vi "refregirator.final.vi"() -> ()   [LabVIEW 2022 SP3]
uses:
  <vilib>/DAQmx/miscellaneous.llb/DAQmx Fill In Error Info.vi
  <vilib>/DAQmx/read.llb/DAQmx Read (Digital Bool 1Line 1Point).vi
  <vilib>/DAQmx/write.llb/DAQmx Write (Digital Bool 1Line 1Point).vi
  <vilib>/DAQmx/read.llb/DAQmx Read (Analog 1D DBL NChan 1Samp).vi
  <vilib>/DAQmx/create/channels.llb/DAQmx Create Channel (DI-Digital Input).vi
  <vilib>/DAQmx/create/channels.llb/DAQmx Create Channel (DO-Digital Output).vi
  <vilib>/DAQmx/create/channels.llb/DAQmx Create Channel (AI-Voltage-Basic).vi
panel:
  out "Cool":bool
  in  "Door Input":tag
  out "Door closed":bool
  in  "Digital Output(Fan)":tag
  out "State":string
  out "Numerical State":dbl
  out "Thermistor temparature":dbl
  out "Outdoor temparature":dbl
  out "Set temparature":dbl
  out "Inside temparature":dbl(knob) scale=0.0..40.0
  out "Outdoor temparature(Celsius)":dbl(knob) scale=0.0..50.0
  in  "stop":bool
  out "Set temparature(Celsius)":dbl(knob) scale=10.0..50.0
  in  "Analog Inputs (Sensors)":tag
  # "Smart Thermo Electric Cooler"
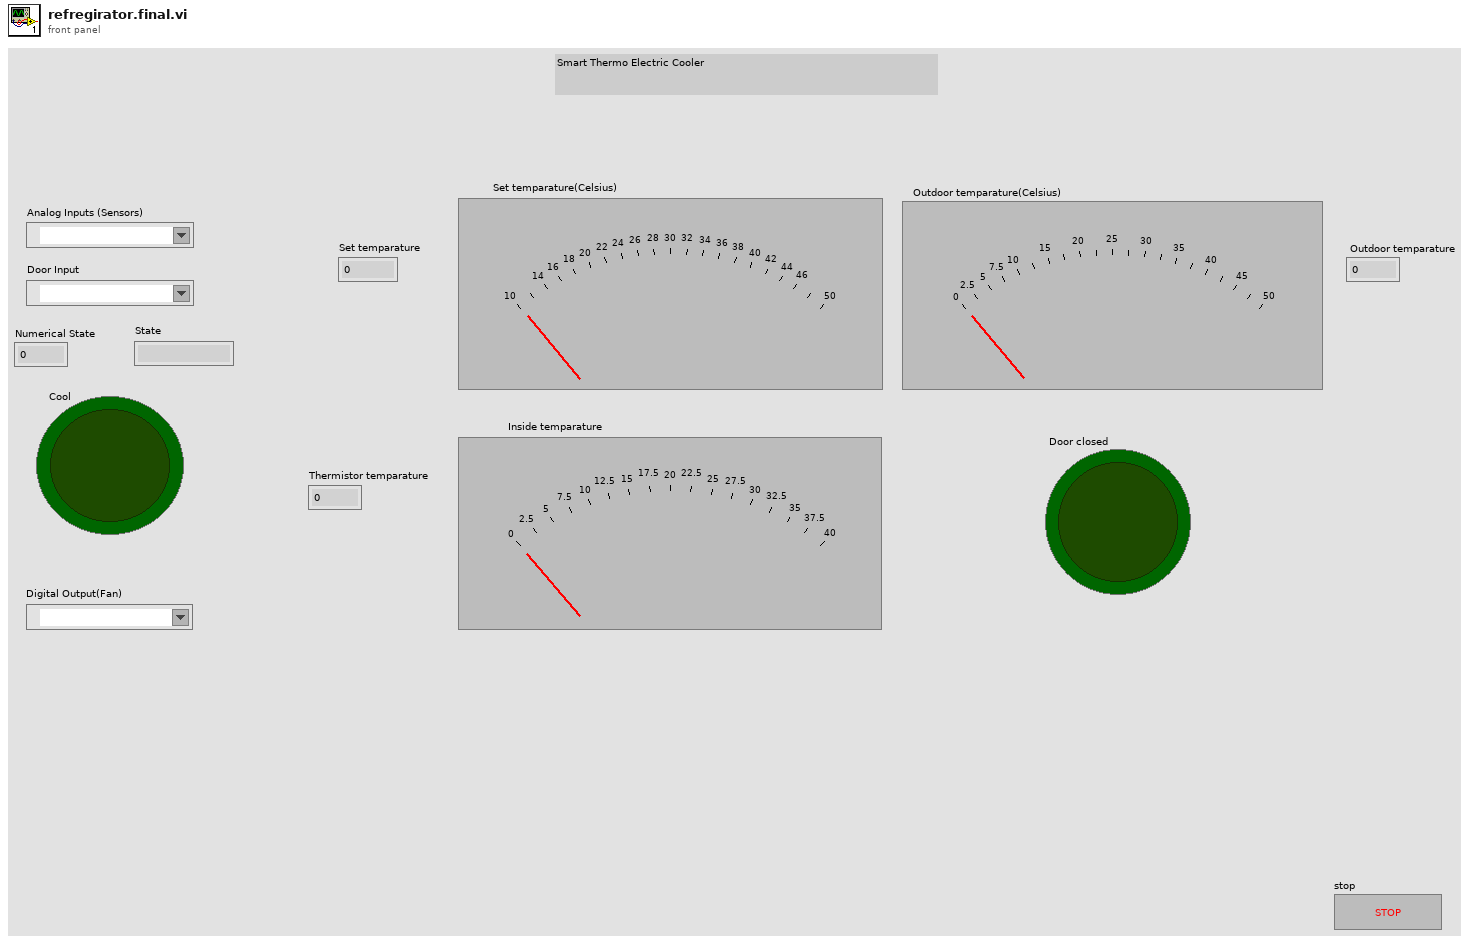
[diagram p1: front panel]
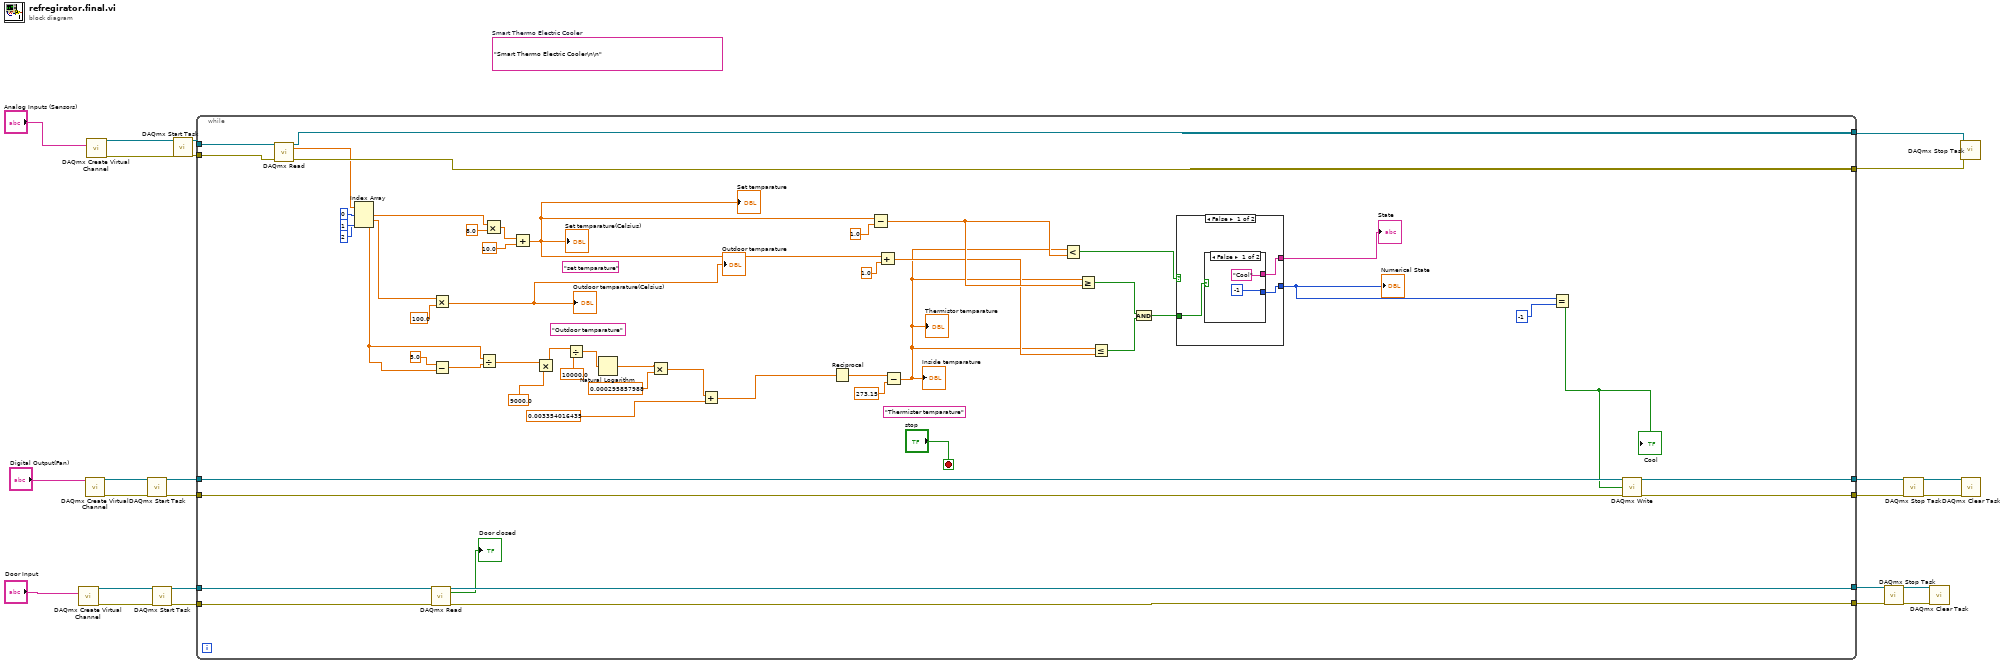
[diagram p0: block diagram]
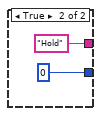
[diagram p2: hidden frame]
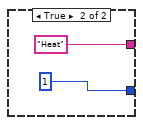
[diagram p3: hidden frame]
diagram:
  (unwired) "Smart Thermo Electric Cooler\n\n"  # Smart Thermo Electric Cooler
  n1 = call-poly <vilib>:"DAQmx Create Virtual Channel.vi"("lines"="Door Input") -> ("task out"=w9:refnum<k21>, "error out"=w8:errorcluster)  [unwired: 13 in]
  n2 = call-poly <vilib>:"DAQmx Create Virtual Channel.vi"("lines"="Digital Output(Fan)") -> ("task out"=w18:refnum<k21>, "error out"=w17:errorcluster)  [unwired: 13 in]
  n3 = call-poly <vilib>:"DAQmx Create Virtual Channel.vi"("physical channels"="Analog Inputs (Sensors)") -> ("task out"=w24:refnum<k21>, "error out"=w23:errorcluster)  [unwired: 13 in]
  n4 = call <vilib>:"DAQmx Start Task.vi"("task/channels in"=w18, "error in"=w17) -> ("task out"=w16:refnum<k21>, "error out"=w15:errorcluster)  [unwired: 12 in]
  n5 = call <vilib>:"DAQmx Start Task.vi"("task/channels in"=w9, "error in"=w8) -> ("task out"=w7:refnum<k21>, "error out"=w6:errorcluster)  [unwired: 12 in]
  n6 = call <vilib>:"DAQmx Start Task.vi"("task/channels in"=w24, "error in"=w23) -> ("task out"=w22:refnum<k21>, "error out"=w21:errorcluster)  [unwired: 12 in]
  n7 = while {
    tunnel: w22 -> [w79]
    tunnel: w21 -> [w78]
    tunnel: [w77] -> w20
    tunnel: [w76] -> w19
    tunnel: w16 -> [w44]
    tunnel: w15 -> [w43]
    tunnel: [w42] -> w14
    tunnel: [w41] -> w13
    tunnel: w7 -> [w33]
    tunnel: w6 -> [w32]
    tunnel: [w31] -> w3
    tunnel: [w30] -> w2
    stop <- "stop" stop-if-true
    (unwired) "Outdoor temparature"
    (unwired) "set temparature"
    (unwired) "Thermister temparature"
    n8 = call-poly <vilib>:"DAQmx Read.vi"("task/channels in"=w79, "error in"=w78) -> ("task out"=w77:refnum<k21>, "data"=w71:dbl[], "error out"=w76:errorcluster)  [unwired: 11 in]
    n9 = Index Array(array=w71, index #1=0 ("index"), index #2=1 ("index"), index #3=2 ("index")) -> (element #1=w67:dbl, element #2=w40:dbl, element #3=w59:dbl)
    n10 = call-poly <vilib>:"DAQmx Read.vi"("task/channels in"=w33, "error in"=w32) -> ("task out"=w31:refnum<k21>, "data"=→"Door closed":bool, "error out"=w30:errorcluster)  [unwired: 11 in]
    n11 = Multiply(x=w40, y=100.0) -> (x*y=→"Outdoor temparature(Celsius)" →"Outdoor temparature":dbl)
    n12 = Subtract(x=5.0 ("y"), y=w59) -> (x-y=w58:dbl)
    n13 = Divide(x=w59, y=w58) -> (x/y=w66:dbl)
    n14 = Multiply(x=w67, y=8.0) -> (x*y=w74:dbl)
    n15 = Add(x=w74, y=10.0) -> (x+y=w28:dbl)
    "Set temparature(Celsius)" <- w28
    "Set temparature" <- w28
    n16 = Multiply(x=w66, y=9000.0) -> (x*y=w34:dbl)
    n17 = Divide(x=w34, y=10000.0) -> (x/y=w36:dbl)
    n18 = Natural Logarithm(1:w36) -> (0:w62:dbl)
    n19 = Multiply(x=w62, y=0.000295857988) -> (x*y=w61:dbl)
    n20 = Add(x=w61, y=0.003354016435) -> (x+y=w35:dbl)
    n21 = Reciprocal(x=w35) -> (1/x=w57:dbl)
    n22 = Subtract(x=w28, y=1.0) -> (x-y=w53:dbl)
    n23 = Add(x=w28, y=1.0) -> (x+y=w52:dbl)
    n24 = Subtract(x=w57, y=273.15) -> (x-y=w27:dbl)
    "Inside temparature" <- w27
    "Thermistor temparature" <- w27
    n25 = Less?(x=w27, y=w53) -> (x < y?=w49:bool)
    n26 = Greater Or Equal?(x=w27, y=w53) -> (x >= y?=w51:bool)
    n27 = Less Or Equal?(x=w27, y=w52) -> (x <= y?=w50:bool)
    n28 = And(x=w51, y=w50) -> (x .and. y?=w48:bool)
    n29 = case shown="False" w49 {
      tunnel: w48 -> [w82 _]
      tunnel: [w81 1] -> w46
      tunnel: [w80 "Heat"] -> w45
      frame False {
        n30 = case shown="False" w82 {
          tunnel: [-1 0] -> w81
          tunnel: ["Cool" "Hold"] -> w80
          frame False {
          }
          frame True {
          }
        }
      }
      frame True {
      }
    }
    "Numerical State" <- w46
    "State" <- w45
    n31 = Equal?(x=w46, y=-1) -> (x = y?=w26:bool)
    "Cool" <- w26
    n32 = call-poly <vilib>:"DAQmx Write.vi"("task/channels in"=w44, "data"=w26, "error in"=w43) -> ("task out"=w42:refnum<k21>, "error out"=w41:errorcluster)  [unwired: 10 in, 1 out]
  }
  n33 = call <vilib>:"DAQmx Stop Task.vi"("task/channels in"=w3, "error in"=w2) -> ("task out"=w5:refnum<k21>, "error out"=w4:errorcluster)  [unwired: 12 in]
  n34 = call <vilib>:"DAQmx Stop Task.vi"("task/channels in"=w14, "error in"=w13) -> ("task out"=w12:refnum<k21>, "error out"=w11:errorcluster)  [unwired: 12 in]
  n35 = call <vilib>:"DAQmx Clear Task.vi"("task in"=w5, "error in"=w4) -> ()  [unwired: 13 in, 1 out]
  n36 = call <vilib>:"DAQmx Stop Task.vi"("task/channels in"=w20, "error in"=w19) -> ()  [unwired: 12 in, 2 out]
  n37 = call <vilib>:"DAQmx Clear Task.vi"("task in"=w12, "error in"=w11) -> ()  [unwired: 13 in, 1 out]
